vi "SetCompressionLevel.vi"(8 "Error In":errorcluster, 10 "Value":i32, 11 "reference in":refnum<class "CompressionDecorator.lvclass">) -> (0 "Error Out":errorcluster, 3 "reference in":refnum<class "CompressionDecorator.lvclass">)   [LabVIEW 2020, in "CompressionDecorator.lvclass"]
uses:
  CompressionDecorator.lvclass
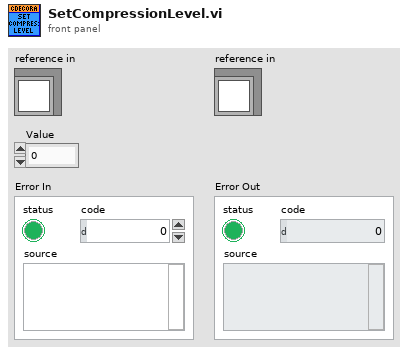
[diagram p1: front panel]
types:
  T1 = typedef "CompressionDecorator.lvclass/ObjectAttributes.ctl" = cluster{"CompLevel":i32}
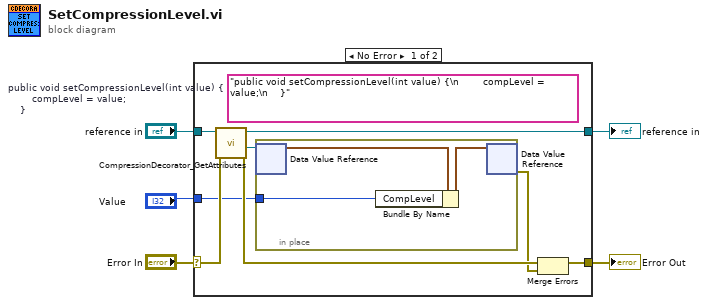
[diagram p0: block diagram]
diagram:
  n1 = case shown="No Error" "Error In" {
    selector: "Error In" -> [w12 w18]
    tunnel: [w11 w18] -> w4
    tunnel: [w10 w17] -> w2
    tunnel: "reference in" -> [w13 w17]
    tunnel: "Value" -> [w6 _]
    frame No Error {
      (unwired) "public void setCompressionLevel(int value) {\n        compLevel = value;\n    }"  # public void setCompressionLevel(int value) {         compLevel = value;     }
      n2 = call "CompressionDecorator_GetAttributes.vi"("error in (no error)"=w12, "reference in"=w13) -> ("error out"=w8:errorcluster, "DataRef"=w9:refnum<data-value>, "reference out"=w10:refnum<class "CompressionDecorator.lvclass">)  [unwired: 6 in, 1 out]
      n3 = in-place {
        in-place-border: w6 -> [w14]
        n4 = in-place-dvr #1(w9) -> (w15:T1)  [unwired: 1 out]
        n5 = Bundle By Name(cluster=w15, "CompLevel"=w14) -> (w16:T1)
        n6 = in-place-dvr #1(w16) -> (w7:errorcluster)  [unwired: 1 out]
      }
      n7 = Merge Errors(w8, w7) -> (w11:errorcluster)
    }
    frame Error {
    }
  }
  "Error Out" <- w4
  "reference in" <- w2
